vi "red ball.vi"(5 "g":dbl=5.0, 6 "L_limit":i32, 7 "jump_heigh":i64=20, 8 "error in":errorcluster, 9 "Jump":bool, 10 "Red_ball":refnum<vi>, 11 "frame in":i32=1) -> (0 "error out":errorcluster, 3 "frame out":i32)   [LabVIEW 2012]
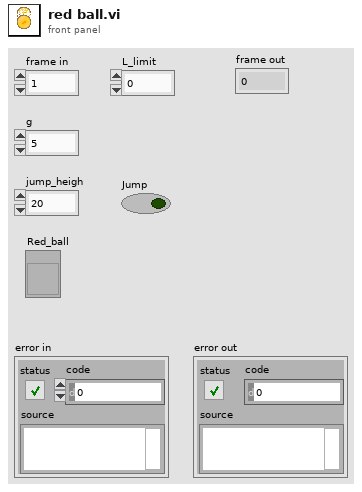
[diagram p1: front panel]
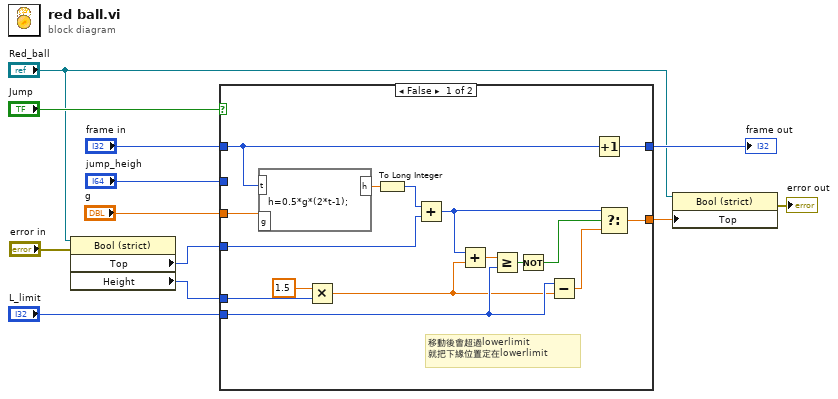
[diagram p0: block diagram]
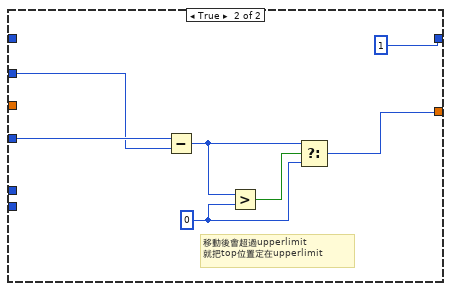
[diagram p2: hidden frame]
diagram:
  n1 = property on="Property Node" class="Bool (strict)"(reference="Red_ball", error in="error in") -> ("Top"=w11:i32, "Height"=w12:u32)  [unwired: 2 out]
  n2 = case shown="False" "Jump" {
    tunnel: w11 -> [w28 w32]
    tunnel: [w27 w34] -> w9
    tunnel: "L_limit" -> [w26 _]
    tunnel: w12 -> [w14 _]
    tunnel: "frame in" -> [w19 _]
    tunnel: [w25 1] -> w6
    tunnel: "g" -> [w18 _]
    tunnel: "jump_heigh" -> [_ w29]
    frame False {
      # "移動後會超過lowerlimit\n就把下緣位置定在lowerlimit"
      n3 = formula code="h=0.5*g*(2*t-1);"("g"=w18, "t"=w19) -> ("h"=w17:dbl)
      n4 = Multiply(x=1.5, y=w14) -> (x*y=w13:dbl)
      n5 = To Long Integer(number=w17) -> (32bit integer=w16:i32)
      n6 = Add(x=w16, y=w28) -> (x+y=w23:i32)
      n7 = Add(x=w23, y=w13) -> (x+y=w24:dbl)
      n8 = Greater Or Equal?(x=w24, y=w26) -> (x >= y?=w21:bool)
      n9 = Not(x=w21) -> (.not. x?=w22:bool)
      n10 = Subtract(x=w26, y=w13) -> (x-y=w20:dbl)
      n11 = Increment(x=w19) -> (x+1=w25:i32)
      n12 = Select(t=w23, s=w22, f=w20) -> (s? t:f=w27:dbl)
    }
    frame True {
      w30 = 0 ("y")
      # "移動後會超過upperlimit\n就把top位置定在upperlimit"
      n13 = Subtract(x=w32, y=w29) -> (x-y=w31:i64)
      n14 = Greater?(x=w31, y=w30) -> (0:w35:bool)
      n15 = Select(t=w31, s=w35, f=w30) -> (s? t:f=w34:i64)
    }
  }
  "frame out" <- w6
  n16 = property on="Property Node" class="Bool (strict)"(reference="Red_ball", "Top"=w9) -> (error out=→"error out":errorcluster)  [unwired: 1 in, 1 out]
